vi "HTS_WRITE_PMC_COMMANDS.vi"(8 "Error IN":errorcluster, 10 "HTS_PMC_COMMANDS":T1, 11 "VISA resource IN":refnum<visa-resource-name>="HTS") -> (0 "Error OUT":errorcluster, 2 "Success?":bool, 3 "VISA resource OUT":refnum<visa-resource-name>)   [LabVIEW 2009]
uses:
  HTS_PMC_COMMAND_LIST.ctl
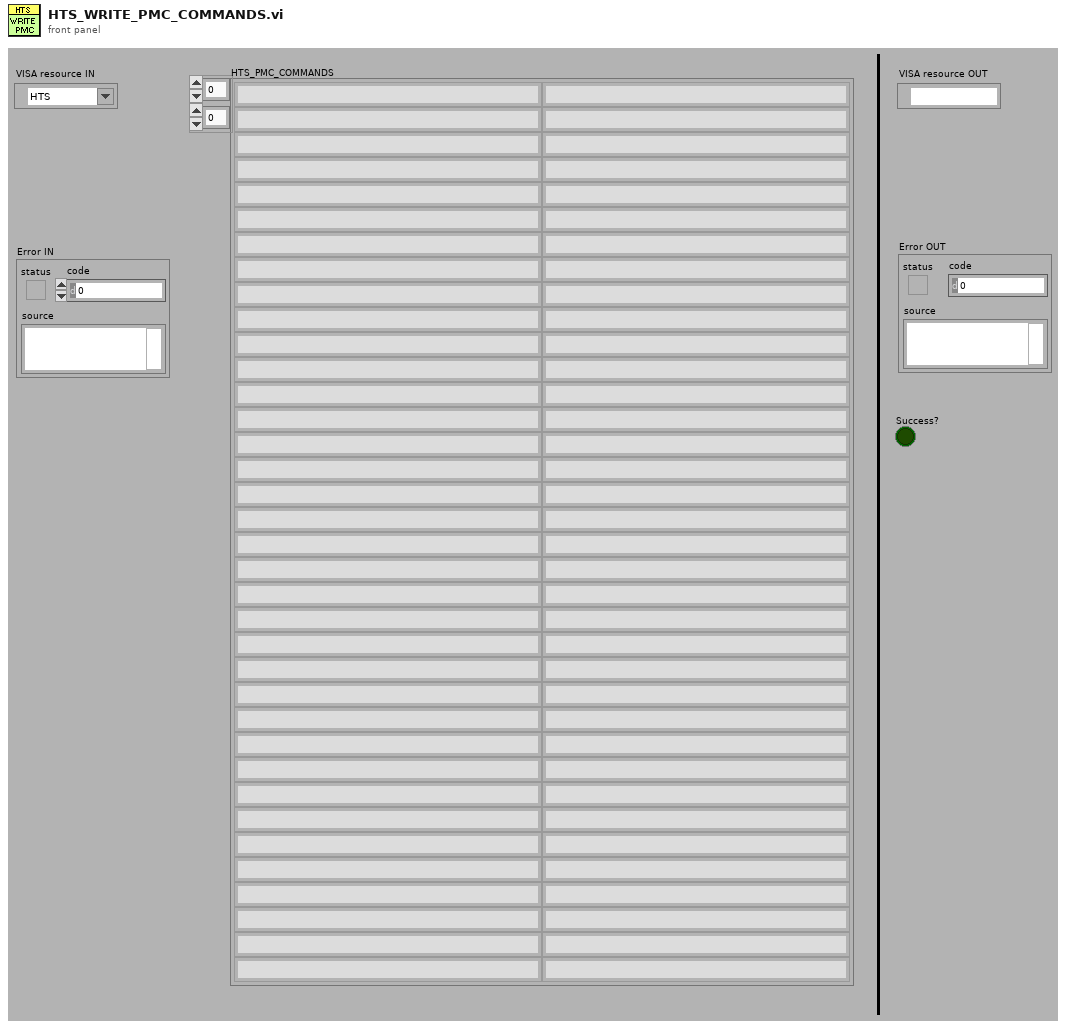
[diagram p1: front panel]
types:
  T1 = typedef "HTS_PMC_COMMAND_LIST.ctl" = string[][]
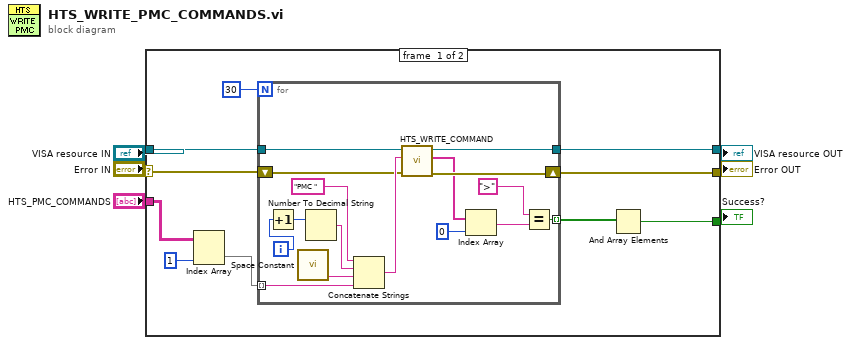
[diagram p0: block diagram]
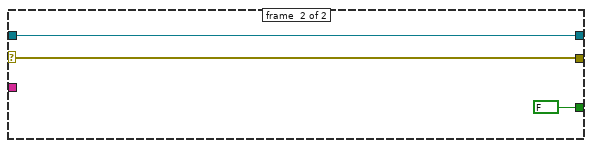
[diagram p2: hidden frame]
diagram:
  n1 = case shown="No Error" "Error IN" {
    selector: "Error IN" -> [w12 w34]
    tunnel: "VISA resource IN" -> [w16 w35]
    tunnel: [w14 w34] -> w5
    tunnel: [w13 w35] -> w4
    tunnel: "HTS_PMC_COMMANDS" -> [w11 _]
    tunnel: [w7 FALSE] -> w1
    frame #0 {
      n2 = Index Array(array=w11, index (col)=1 ("disabled index (col)")) -> (element=w9:string[])  [unwired: 1 in]
      n3 = for {
        N: 30 -> [_]
        tunnel: w16 -> [w32]
        tunnel: [w17] -> w8 mode=indexing
        shift-right: [w27] -> w14
        shift-left: w12 -> [w28]
        tunnel: [w24] -> w13
        tunnel: w9 -> [w22] mode=indexing
        i -> [w26]
        n4 = Increment(x=w26) -> (x+1=w25:i32)
        n5 = call <vilib>:"Space Constant.vi"() -> ("String"=w23:string)
        n6 = Number To Decimal String(number=w25) -> (decimal integer string=w31:string)  [unwired: 1 out]
        n7 = Concatenate Strings("PMC ", w31, w23, w22) -> (w29:string)
        n8 = call "HTS_WRITE_COMMAND.vi"("Error IN"=w28, "Command"=w29, "VISA resource IN"=w32) -> ("Error OUT"=w27:errorcluster, "RESPONSE"=w20:string[], "VISA resource OUT"=w24:refnum<visa-resource-name>)  [unwired: 6 out]
        n9 = Index Array(array=w20, index=0) -> (element=w21:string)
        n10 = Equal?(x=">", y=w21) -> (x = y?=w17:bool)
      }
      n11 = And Array Elements(Boolean array=w8) -> (logical AND=w7:bool)
    }
    frame #1 {
    }
  }
  "Error OUT" <- w5
  "VISA resource OUT" <- w4
  "Success?" <- w1
